vi "image_info_service.vi"(11 "Image":T2) -> (2 "Image Name":string, 3 "size":T1)   [LabVIEW 2021]
uses:
  <vilib>/vision/Image Controls.llb/IMAQ Image.ctl
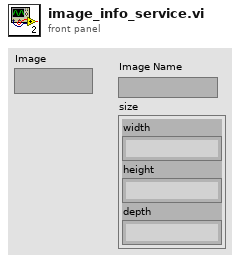
[diagram p1: front panel]
types:
  T1 = cluster{"width":string, "height":string, "depth ":string}
  T2 = typedef "IMAQ Image.ctl" = refnum<image>
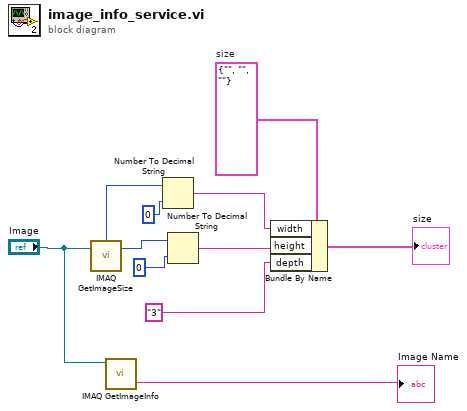
[diagram p0: block diagram]
diagram:
  w7 = T1 {"width"="", "height"="", "depth "=""}  # size
  n1 = call "IMAQ GetImageSize"("Image"="Image") -> ("Y Resolution"=w11:i32, "X Resolution"=w8:i32)  [unwired: 3 in, 1 out]
  n2 = call "IMAQ GetImageInfo"("Image"="Image") -> ("Image Name"=→"Image Name":string)  [unwired: 3 in, 7 out]
  n3 = Number To Decimal String(number=w8, width (-)=i16 0) -> (decimal integer string=w4:string)
  n4 = Number To Decimal String(number=w11, width (-)=i16 0) -> (decimal integer string=w5:string)
  n5 = Bundle By Name(cluster=w7, "width"=w4, "height"=w5, "depth"="3") -> (→"size":T1)
